vi "ReadADC.vi"(8 "error in (no error)":errorcluster, 10 "ADC Channel":dbl, 11 "Cypress in":refnum<class "Cypress.lvclass">) -> (0 "error out":errorcluster, 3 "Cypress out":refnum<class "Cypress.lvclass">)   [LabVIEW 2020, in "Cypress.lvclass"]
uses:
  Cypress.lvclass
  Abstract/Serial Device/Serial Device.lvclass
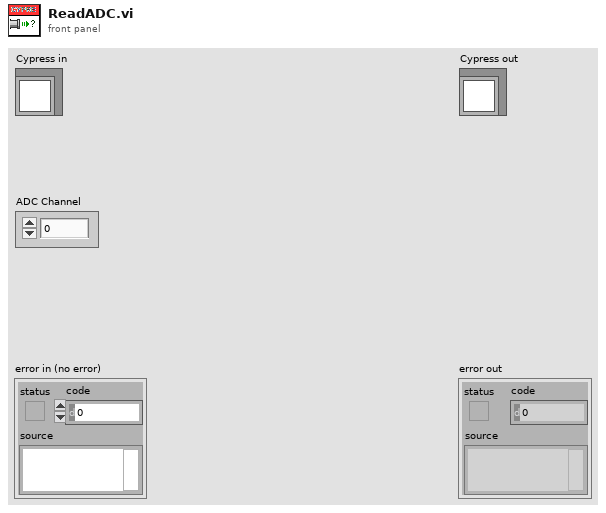
[diagram p1: front panel]
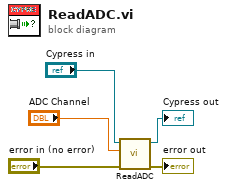
[diagram p0: block diagram]
diagram:
  n1 = call-parent "ReadADC.vi"("error in (no error)"="error in (no error)", "ADC Channel"="ADC Channel", "Serial Device in"="Cypress in") -> ("error out"=→"error out":errorcluster, "Serial Device out"=→"Cypress out":refnum<class "Cypress.lvclass">)  [unwired: 7 in]
